vi "Kill-VI.vi"() -> ()   [LabVIEW 2013]
panel:
  in  "VI Name to kill":string
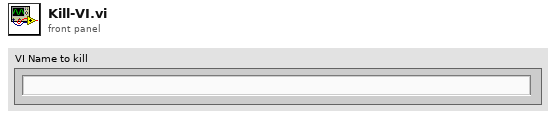
[diagram p1: front panel]
types:
  T1 = enum32{"Bad", "Idle", "Run top level", "Running"}
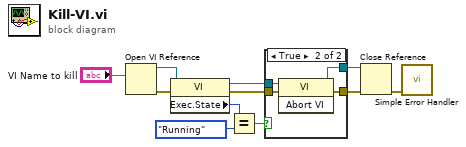
[diagram p0: block diagram]
diagram:
  n1 = Open VI Reference(vi path="VI Name to kill") -> (vi reference=w10:refnum<vi>, error out=w11:errorcluster)  [unwired: 5 in]
  n2 = property class="VI"(reference=w10, error in=w11) -> (reference out=w7:refnum<vi>, error out=w5:errorcluster, "Exec.State"=w9:T1)
  n3 = Equal?(x=w9, y=T1."Running" ("Execution:State")) -> (x = y?=w1:bool)
  n4 = case shown="True" w1 {
    tunnel: w7 -> [w13 w17]
    tunnel: [w13 w16] -> w6
    tunnel: w5 -> [w12 w15]
    tunnel: [w12 w14] -> w4
    frame False {
    }
    frame True {
      n5 = invoke class="VI" method="Abort VI"(reference=w17, error in=w15) -> (reference out=w16:refnum<vi>, error out=w14:errorcluster)  [unwired: 1 in, 1 out]
    }
  }
  n6 = Close Reference(reference=w6, error in (no error)=w4) -> (error out=w2:errorcluster)
  n7 = call <vilib>:"Simple Error Handler.vi"("error in (no error)"=w2) -> ()  [unwired: 4 in, 5 out]
